vi "qHIN.vi"(0 "System no.":i32=1 min=1 max=4 step=1, 2 "Axes to query":string[](array[string]), 3 "All axes?":bool, 4 "Axis identifier?":bool=TRUE, 5 "error in":errorcluster) -> (14 "HID control status?":bool[](array[boolean]), 19 "error out":errorcluster)   [LabVIEW 2026]
doc: "Returns current HID control status of queried axes of the controller. See controller user manual for details.\n\nAll systems: If All axes? = TRUE, then Axis identifier? can be FALSE\nC-867:"
panel:
  # "Returns current HID control status of queried axes of the controller."
  # "If all axes: use"
  # "Query"
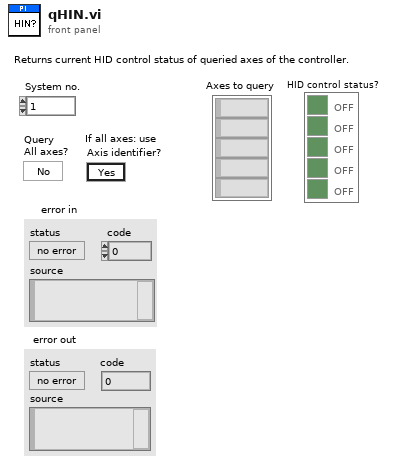
[diagram p1: front panel]
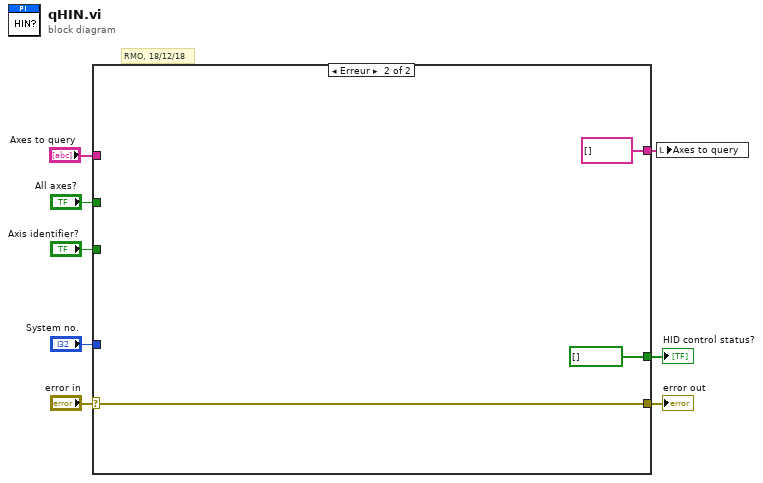
[diagram p0: block diagram]
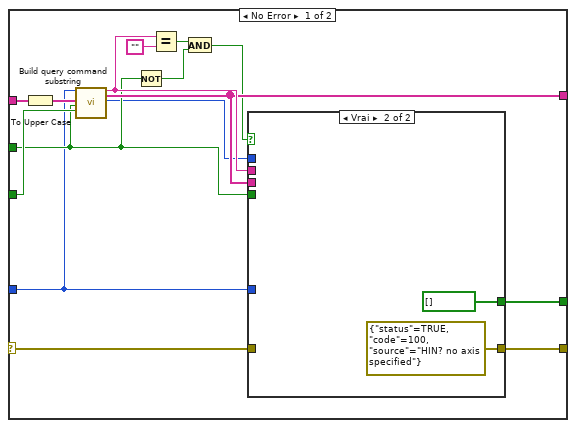
[diagram p2: hidden frame]
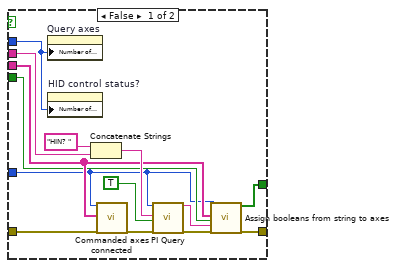
[diagram p3: hidden frame]
diagram:
  # "RMO, 18/12/18"
  n1 = case shown="Erreur" "error in" {
    selector: "error in" -> [w12 w40]
    tunnel: [w23 bool[] [] ("Booleans")] -> w8
    tunnel: "Axes to query" -> [w22 _]
    tunnel: [w10 w40] -> w6
    tunnel: "Axis identifier?" -> [w19 _]
    tunnel: "System no." -> [w11 _]
    tunnel: [w17 string[] [] ("Axes to query out")] -> w3
    tunnel: "All axes?" -> [w16 _]
    frame No Error {
      n2 = To Upper Case(1:w22) -> (0:w20:string[])
      n3 = call "Build query command substring.vi"("System no."=w11, "Axes to query in"=w20, "Query\nAll axes?"=w16, "For all axes: use\nAxis identifier?"=w19) -> ("Command substring"=w18:string, "Axes to query out"=w17:string[], "Number of rows"=w13:u32)  [unwired: 2 in, 11 out]
      n4 = Not(x=w16) -> (.not. x?=w14:bool)
      n5 = Equal?(x=w18, y="" ("x")) -> (x = y?=w15:bool)
      n6 = And(x=w15, y=w14) -> (x .and. y?=w9:bool)
      n7 = case shown="Vrai" w9 {
        tunnel: [w34 bool[] [] ("Booleans")] -> w23
        tunnel: w18 -> [w33 _]
        tunnel: w17 -> [w32 _]
        tunnel: w16 -> [w31 _]
        tunnel: w13 -> [w30 _]
        tunnel: w12 -> [w28 _]
        tunnel: w11 -> [w26 _]
        tunnel: [w24 errorcluster {"status"=TRUE, "code"=100, "source"="HIN? no axis specified"} ("error out")] -> w10
        frame False {
          n8 = property on="Query axes" class="Tabl (strict)"("Number of Rows"=w30) -> ()  [unwired: 2 in, 2 out]
          n9 = property on="HID control status?" class="Tabl (strict)"("Number of Rows"=w30) -> ()  [unwired: 2 in, 2 out]
          n10 = Concatenate Strings("HIN? ", w33) -> (w35:string)
          n11 = call "Commanded axes connected.vi"("System no."=w26, "Commanded axes"=w32, "error in"=w28) -> ("error out"=w29:errorcluster)  [unwired: 1 in, 15 out]
          n12 = call "PI Query.vi"("System no."=w26, "String to send"=w35, "Attach termination char.?"=TRUE ("Attach Linefeed?"), "error in"=w29) -> ("String read"=w25:string, "error out"=w27:errorcluster)  [unwired: 3 in, 11 out]
          n13 = call "Assign booleans from string to axes.vi"("System no."=w26, "Queried axes"=w32, "All axes queried?"=w31, "Input String"=w25, "error in"=w27) -> ("Booleans"=w34:bool[], "error out"=w24:errorcluster)  [unwired: 13 out]
        }
        frame True {
        }
      }
    }
    frame Error {
    }
  }
  "error out" <- w6
  "HID control status?" <- w8
  n14 = local write "Axes to query"(w3) -> ()
